vi "hmi_update_software_list.vi"(5 "hmi_references":T1, 7 "post_installer []":refnum<class "lv-post-installer.lvclass">[](array[class]), 8 "error in (no error)":errorcluster) -> (0 "error out":errorcluster)   [LabVIEW 2015, in "lv-post-installer-interface.lvlib"]
uses:
  lv-post-installer-interface.lvlib
  lv-post-installer/public/classes/lv-post-installer/lv-post-installer.lvclass
  _controls/hmi_references.ctl
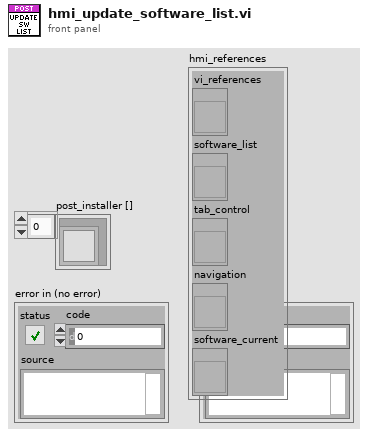
[diagram p1: front panel]
types:
  T1 = typedef "lv-post-installer-interface.lvlib/hmi_references.ctl" = cluster{"vi_references":refnum<vi>, "software_list":refnum<vi>, "tab_control":refnum<vi>, "navigation":refnum<vi>, "software_current":refnum<vi>}
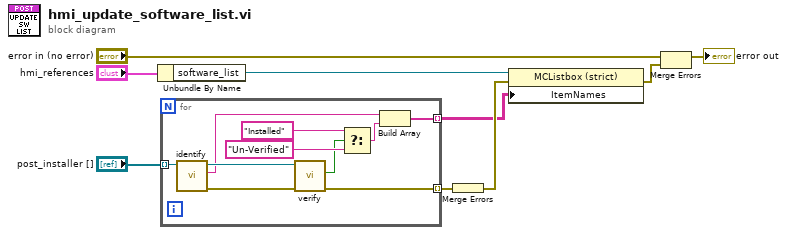
[diagram p0: block diagram]
diagram:
  n1 = Unbundle By Name("hmi_references") -> ("software_list"=w4:refnum<vi>)
  n2 = for {
    tunnel: [w15] -> w3 mode=indexing
    tunnel: [w16] -> w5 mode=indexing
    tunnel: "post_installer []" -> [w11] mode=indexing
    n3 = call-dynamic "identify.vi"("plugin_interface in"=w11) -> ("error out"=w12:errorcluster, "identifier"=w10:string, "plugin_interface out"=w14:refnum<class "lv-post-installer.lvclass">)  [unwired: 8 in]
    n4 = call-dynamic "verify.vi"("error in (no error)"=w12, "plugin_interface in"=w14) -> ("error out"=w15:errorcluster, "installed?"=w13:bool)  [unwired: 7 in, 1 out]
    n5 = Select(t="Installed", s=w13, f="Un-Verified") -> (s? t:f=w17:string)
    n6 = Build Array(w10, w17) -> (w16:string[])
  }
  n7 = Merge Errors(w3) -> (w6:errorcluster)
  n8 = property on="Property Node" class="MCListbox (strict)"(reference=w4, error in=w6, "ItemNames"=w5) -> (error out=w9:errorcluster)  [unwired: 1 out]
  n9 = Merge Errors("error in (no error)", w9) -> (→"error out":errorcluster)
